vi "Message Based DAQ.vi"() -> ()   [LabVIEW 2014]
uses:
  <vilib>/Utility/error.llb/DialogType.ctl
  vilib/Message/Msg Post UI Message.vi
  vilib/Message/Msg Post Queue Message.vi
  vilib/Message/Msg Send Queue Message.vi
panel:
  in  "File Path":path
  in  "Acquire Data":bool
  in  "Log Data":bool
  in  "File Comment":string
  in  "DAQ Parameters":T1={"physical channels"="", "maximum value"=5.0, "minimum value"=-5.0, "rate"=1000.0, "read period"=0.5} {"read period" format="%0.2f"; "rate" format="%0.2f"; "minimum value" format="%0.2f"; "maximum value" format="%0.2f"}
  out "Waveform Chart":waveform(dbl)(graph)
  in  "quit":bool
  # "V"
  # "V"
  # "Hz"
  # "s"
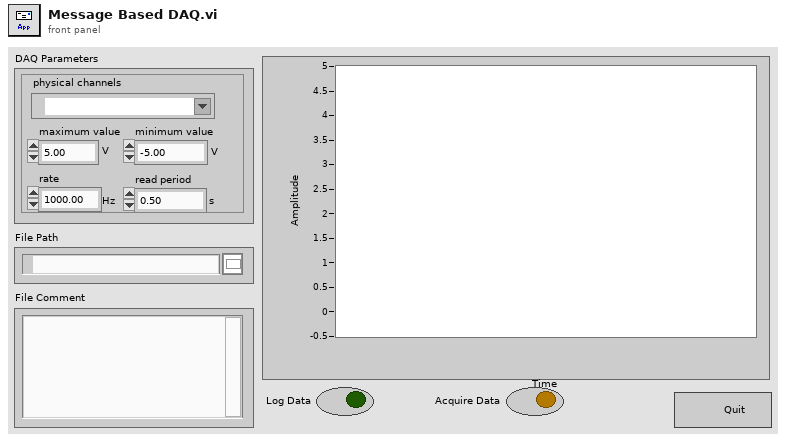
[diagram p1: front panel]
types:
  T1 = cluster{"physical channels":tag, "maximum value":dbl, "minimum value":dbl, "rate":dbl, "read period":dbl}
  T2 = typedef "DialogType.ctl" = u16
  T3 = enum16{"Left Button", "Center Button", "Right Button", "Window Close"}
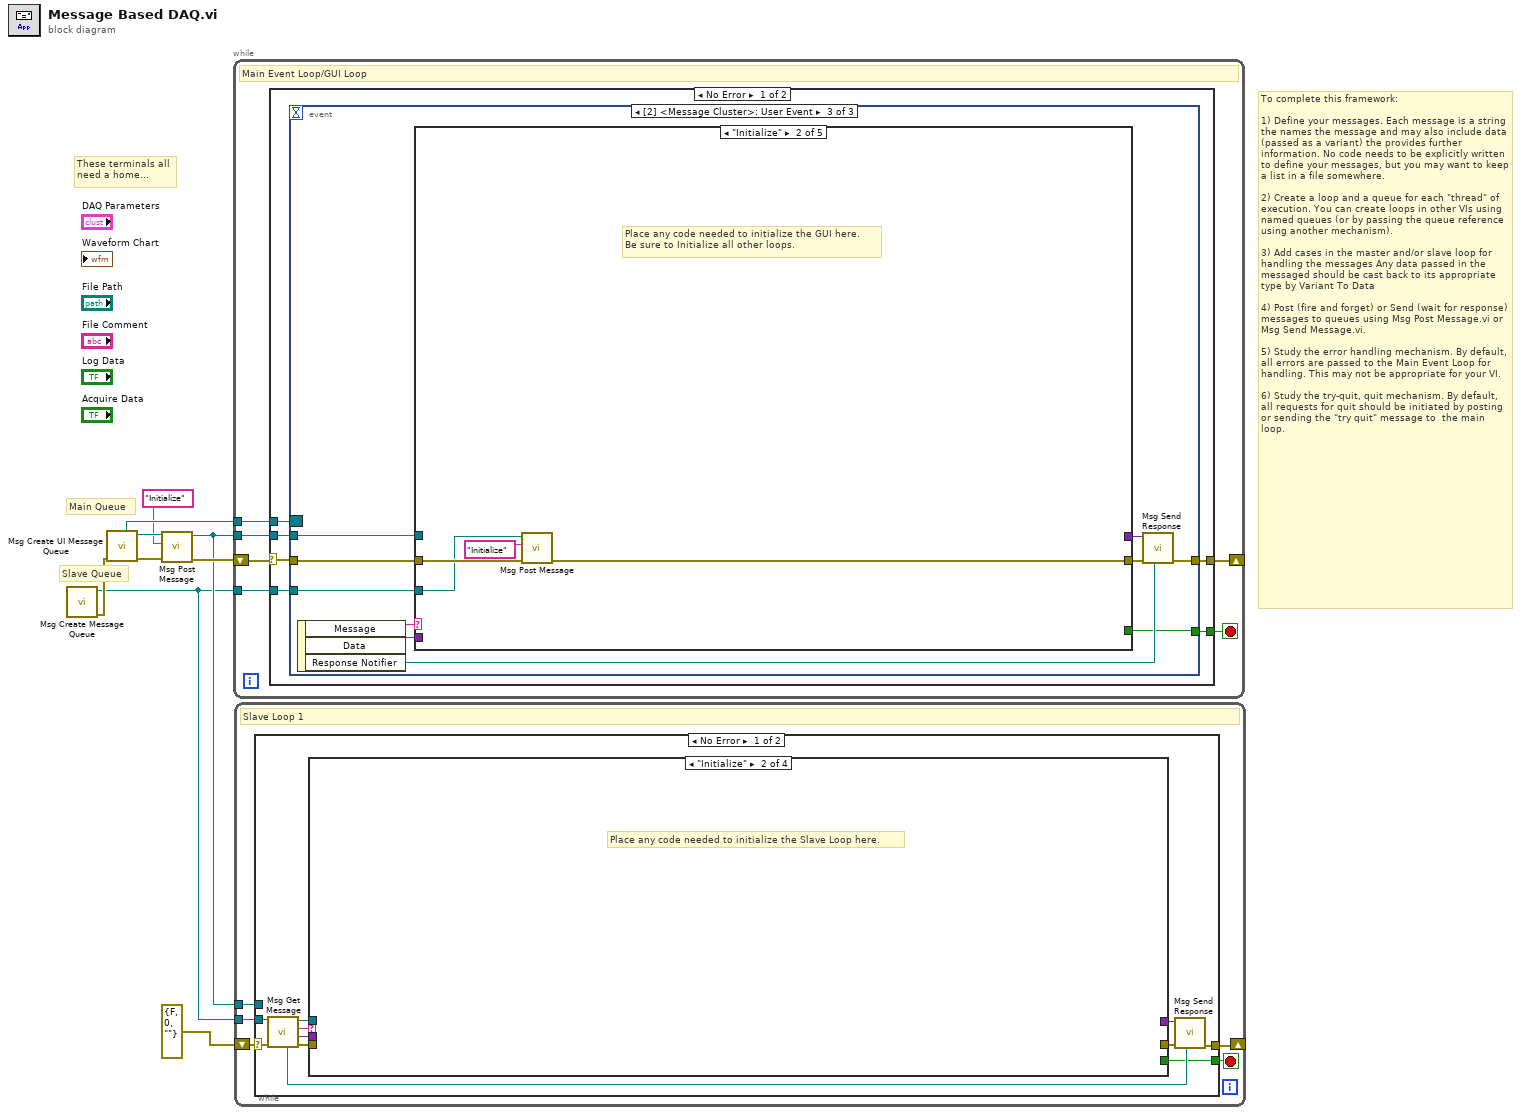
[diagram p0: block diagram]
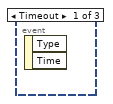
[diagram p2: hidden frame]
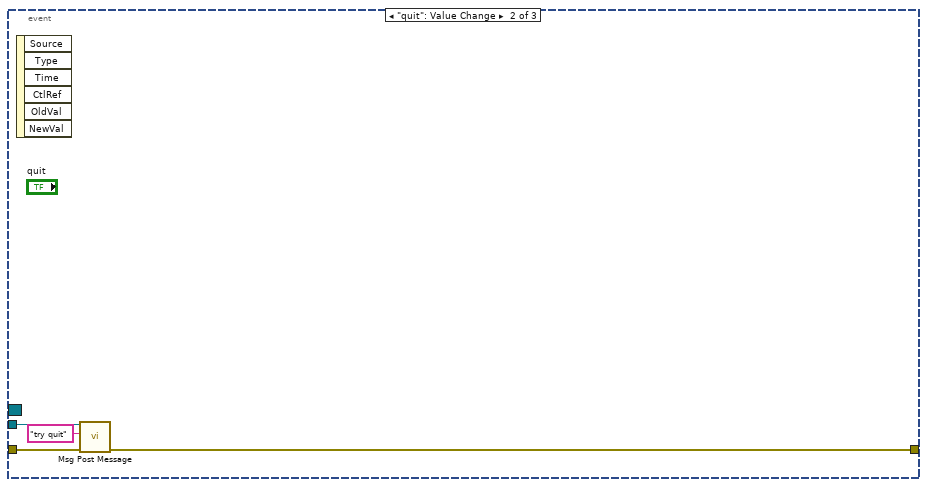
[diagram p3: hidden frame]
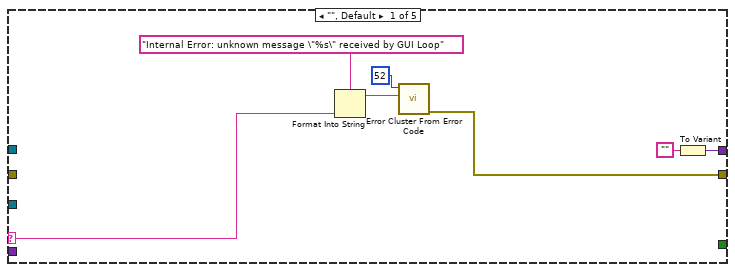
[diagram p4: hidden frame]
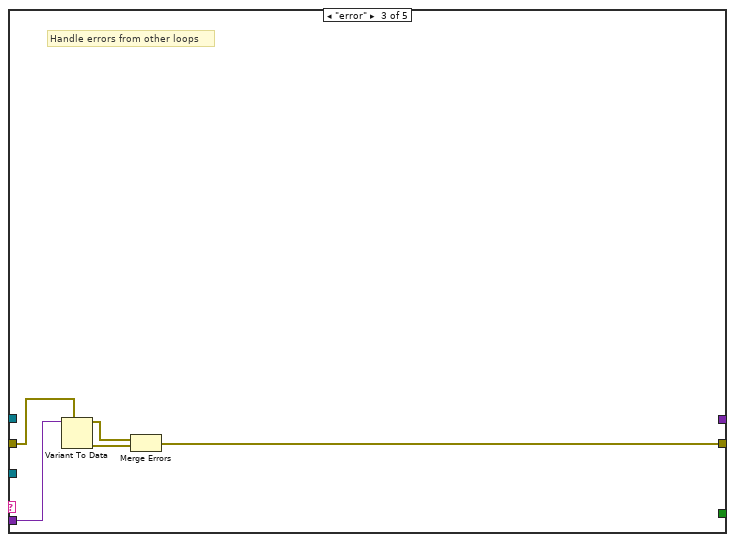
[diagram p5: hidden frame]
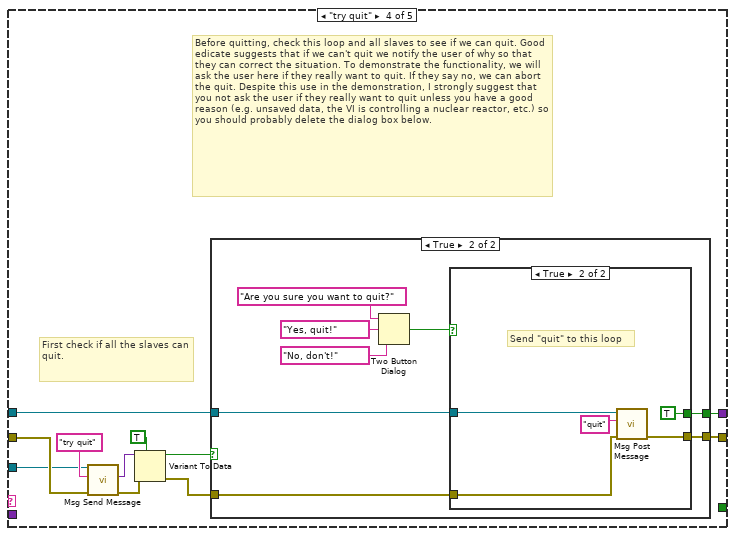
[diagram p6: hidden frame]
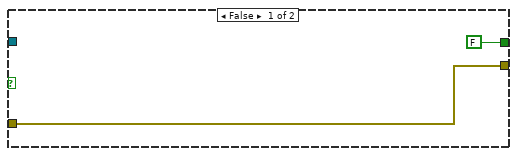
[diagram p7: hidden frame]
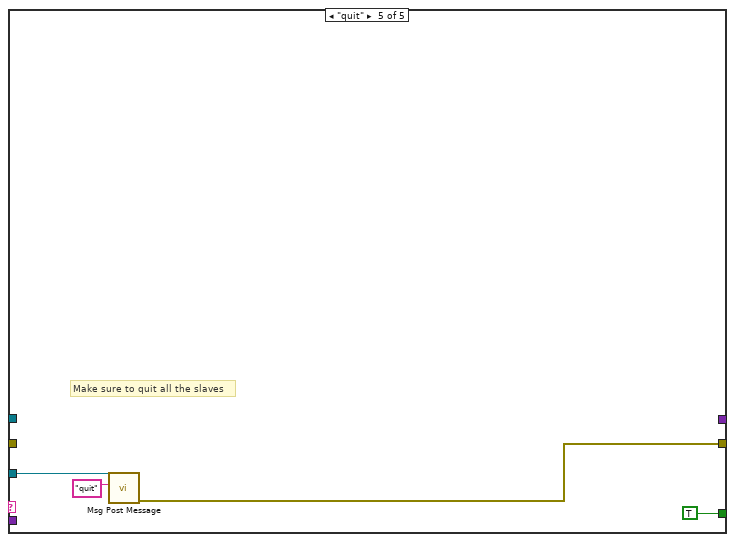
[diagram p9: hidden frame]
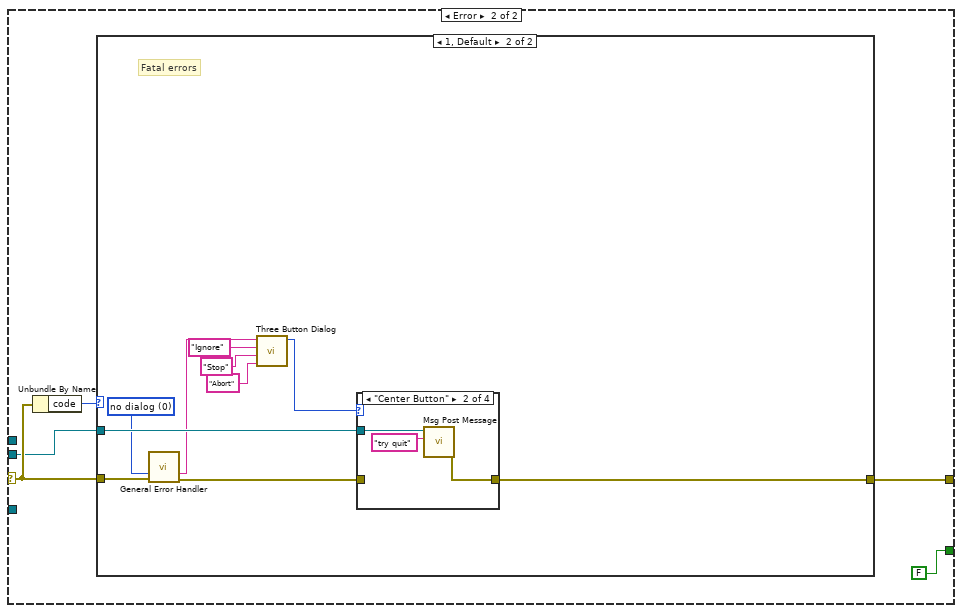
[diagram p10: hidden frame]
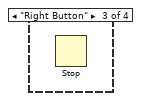
[diagram p13: hidden frame]
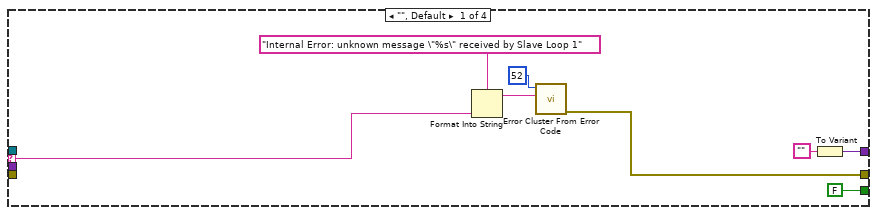
[diagram p15: hidden frame]
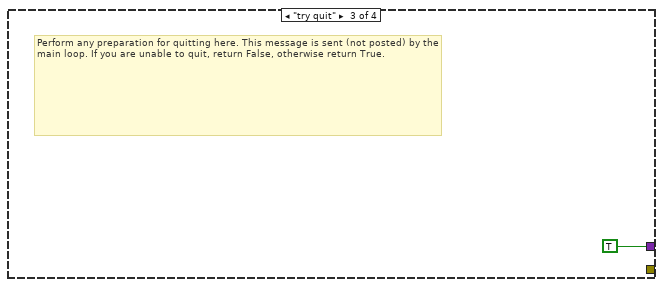
[diagram p16: hidden frame]
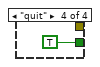
[diagram p17: hidden frame]
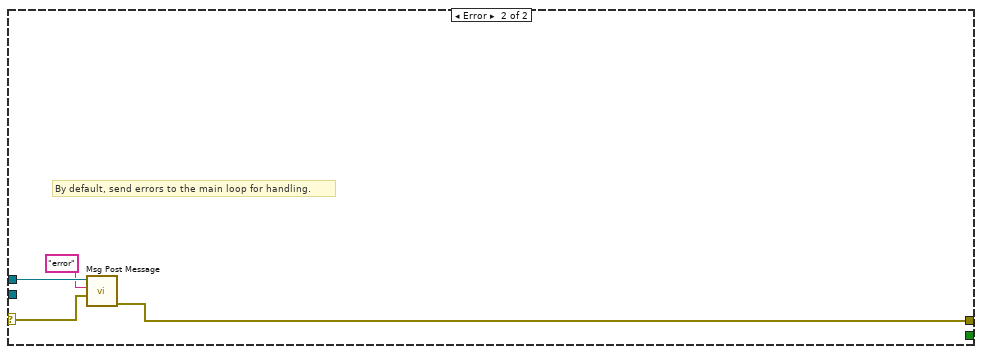
[diagram p18: hidden frame]
diagram:
  # "These terminals all\nneed a home..."
  # "To complete this framework:\n\n1) Define your messages. Each message is a string the names the message and may also include data (passed as a variant) the provides further information. No code needs to be explicitly written to define your messages, but you may want to keep a list in a file somewhere.\n\n2) Create a loop and a queue for each \"thread\" of execution. You can create loops in other VIs using named queues (or by passing the queue reference using another mechanism).\n\n3) Add cases in the master and/or slave loop for handling the messages Any data passed in the messaged should be cast back to its appropriate type by Variant To Data\n\n4) Post (fire and forget) or Send (wait for response) messages to queues using Msg Post Message.vi or Msg Send Message.vi.\n\n5) Study the error handling mechanism. By default, all errors are passed to the Main Event Loop for handling. This may not be appropriate for your VI.\n\n6) Study the try-quit, quit mechanism. By default, all requests for quit should be initiated by posting or sending the \"try quit\" message to  the main loop."
  # "Main Queue"
  # "Slave Queue"
  n1 = call "Msg Create Message Queue.vi"() -> ("error out"=w5:errorcluster, "queue out"=w2:refnum<queue>)  [unwired: 7 in, 1 out]
  n2 = call "Msg Create UI Message Queue.vi"("error in (no error)"=w5) -> ("error out"=w6:errorcluster, "user event"=w8:refnum<user-event>, "Event Registration Refnum out"=w9:refnum<event-registration>)  [unwired: 6 in]
  n3 = call-poly "Msg Post Message.vi"("error in (no error)"=w6, "Message"="Initialize", "user event"=w8) -> ("error out"=w4:errorcluster, "user event out"=w3:refnum<user-event>)  [unwired: 4 in, 1 out]
  n4 = while {
    tunnel: w9 -> [w14]
    shift-right: [w12] -> _
    shift-left: w4 -> [w10]
    tunnel: w3 -> [w13]
    tunnel: w2 -> [w11]
    stop <- w15 stop-if-true
    # "Main Event Loop/GUI Loop"
    n5 = case shown="No Error" w10 {
      selector: w10 -> [w16 w85]
      tunnel: [w21 FALSE] -> w15
      tunnel: w14 -> [w20 _]
      tunnel: w13 -> [w19 w84]
      tunnel: [w18 w83] -> w12
      tunnel: w11 -> [w17 _]
      frame No Error {
        n6 = event shown="[2] <Message Cluster>: User Event" {
          selector: w20 -> [_ _ _]
          dyn-events: _ -> [_ _ _]
          timeout: _ -> [_ _ _]
          tunnel: [_ _ w26] -> w21
          tunnel: w19 -> [_ w25 w27]
          tunnel: w16 -> [_ w24 w32]
          tunnel: [_ w23 w30] -> w18
          tunnel: w17 -> [_ _ w28]
          event Timeout {
            n7 = event-data() -> ()  [unwired: 1 in, 2 out]
          }
          event "quit": Value Change {
            n8 = event-data() -> ()  [unwired: 1 in, 6 out]
            n9 = call-poly "Msg Post Message.vi"("error in (no error)"=w24, "Message"="try quit", "user event"=w25) -> ("error out"=w23:errorcluster)  [unwired: 4 in, 2 out]
          }
          event User Event {
            n10 = event-data() -> ("Message"=w35:string, "Data"=w29:variant, "Response Notifier"=w33:refnum<notifier>)  [unwired: 1 in]
            n11 = case shown="\"Initialize\"" w35 {
              selector: w35 -> [w40 _ _ _ _]
              tunnel: [w41 _ _ w55 _] -> w34
              tunnel: w32 -> [_ w46 w50 w62 _]
              tunnel: [w36 w43 w47 w56 w79] -> w31
              tunnel: w29 -> [_ _ w51 _ _]
              tunnel: w28 -> [_ w45 _ w53 w80]
              tunnel: w27 -> [_ _ _ w57 _]
              tunnel: [_ _ _ _ TRUE] -> w26
              frame "", Default {
                n12 = Format Into String(format string="Internal Error: unknown message \"%s\" received by GUI Loop" ("error message (\"\")"), w40) -> (resulting string=w37:string)  [unwired: 2 in, 1 out]
                n13 = call <vilib>:"Error Cluster From Error Code.vi"("error message (\"\")"=w37, "error code (0)"=52) -> ("error out"=w36:errorcluster)  [unwired: 7 in]
                n14 = To Variant(anything="") -> (Variant=w41:variant)
              }
              frame "Initialize" {
                # "Place any code needed to initialize the GUI here. \nBe sure to Initialize all other loops."
                n15 = call-poly "Msg Post Message.vi"("error in (no error)"=w46, "Message"="Initialize", "queue"=w45) -> ("error out"=w43:errorcluster)  [unwired: 4 in, 2 out]
              }
              frame "error" {
                # "Handle errors from other loops"
                n16 = Variant To Data(type=w50, Variant=w51) -> (data=w49:errorcluster, error out=w48:errorcluster)  [unwired: 1 in]
                n17 = Merge Errors(w49, w48) -> (w47:errorcluster)
              }
              frame "try quit" {
                # "Before quitting, check this loop and all slaves to see if we can quit. Good edicate suggests that if we can't quit we notify the user of why so that they can correct the situation. To demonstrate the functionality, we will ask the user here if they really want to quit. If they say no, we can abort the quit. Despite this use in the demonstration, I strongly suggest that you not ask the user if they really want to quit unless you have a good reason (e.g. unsaved data, the VI is controlling a nuclear reactor, etc.) so you should probably delete the dialog box below."
                # "First check if all the slaves can quit."
                n18 = call-poly "Msg Send Message.vi"("error in (no error)"=w62, "Message"="try quit", "queue"=w53) -> ("error out"=w60:errorcluster, "response"=w54:variant)  [unwired: 3 in, 2 out]
                n19 = Variant To Data(error in=w60, type=TRUE, Variant=w54) -> (data=w52:bool, error out=w58:errorcluster)
                n20 = case shown="True" w52 {
                  tunnel: w58 -> [w64 w71]
                  tunnel: w57 -> [_ w72]
                  tunnel: [w64 w70] -> w56
                  tunnel: [FALSE w69] -> w55
                  frame False {
                  }
                  frame True {
                    n21 = Two Button Dialog(message="Are you sure you want to quit?", 1:"No, don't!" ("T button name (\"OK\")"), 2:"Yes, quit!" ("T button name (\"OK\")")) -> (T button?=w65:bool)
                    n22 = case shown="True" w65 {
                      tunnel: w72 -> [_ w78]
                      tunnel: w71 -> [w73 w76]
                      tunnel: [w73 w75] -> w70
                      tunnel: [_ TRUE] -> w69
                      frame False {
                      }
                      frame True {
                        # "Send \"quit\" to this loop"
                        n23 = call-poly "Msg Post Message.vi"("error in (no error)"=w76, "Message"="quit", "user event"=w78) -> ("error out"=w75:errorcluster)  [unwired: 4 in, 2 out]
                      }
                    }
                  }
                }
              }
              frame "quit" {
                # "Make sure to quit all the slaves"
                n24 = call-poly "Msg Post Message.vi"("Message"="quit", "queue"=w80) -> ("error out"=w79:errorcluster)  [unwired: 5 in, 2 out]
              }
            }
            n25 = call "Msg Send Response.vi"("Response Notifier"=w33, "error in (no error)"=w31, "response"=w34) -> ("error out"=w30:errorcluster)  [unwired: 6 in]
          }
        }
      }
      frame Error {
        n26 = Unbundle By Name(w85) -> ("code"=w86:i32)
        n27 = case shown="1, Default" w86 {
          tunnel: w85 -> [_ w97]
          tunnel: w84 -> [_ w96]
          tunnel: [_ w94] -> w83
          frame 0 {
            # "Ignore these errors"
          }
          frame 1, Default {
            w93 = T2 0 items=["no dialog", "OK message", "continue or stop message", "OK message + warnings", "continue/stop + warnings"] ("type of dialog (OK msg:1)")
            # "Fatal errors"
            n28 = call <vilib>:"General Error Handler.vi"("type of dialog (OK msg:1)"=w93, "error in (no error)"=w97) -> ("message"=w92:string, "error out"=w95:errorcluster)  [unwired: 9 in, 3 out]
            n29 = call <vilib>:"Three Button Dialog.vi"("Right Button Text (\"Cancel\")"="Abort" ("Right Button Text (\"Cancel\")"), "Center Button Text (\"No\")"="Stop" ("Center Button Text (\"No\")"), "Left Button Text (\"Yes\")"="Ignore" ("Left Button Text (\"Yes\")"), "message"=w92) -> ("Which Button?"=w88:T3)  [unwired: 7 in]
            n30 = case shown="\"Center Button\"" w88 {
              tunnel: w96 -> [_ w100 _ _]
              tunnel: w95 -> [_ _ _ _]
              tunnel: [_ w98 _ _] -> w94
              frame "Left Button", Default {
              }
              frame "Center Button" {
                n31 = call-poly "Msg Post Message.vi"("Message"="try quit", "user event"=w100) -> ("error out"=w98:errorcluster)  [unwired: 5 in, 2 out]
              }
              frame "Right Button" {
                n32 = Stop() -> ()  [unwired: 1 in]
              }
              frame "Window Close" {
              }
            }
          }
        }
      }
    }
  }
  n33 = while {
    tunnel: w3 -> [w101]
    tunnel: w2 -> [w105]
    shift-right: [w104] -> _
    shift-left: errorcluster {"status"=FALSE, "code"=0, "source"=""} ("error out") -> [w102]
    stop <- w103 stop-if-true
    # "Slave Loop 1"
    n34 = case shown="No Error" w102 {
      selector: w102 -> [w106 w128]
      tunnel: w105 -> [w116 _]
      tunnel: [w110 w127] -> w104
      tunnel: [w107 _] -> w103
      tunnel: w101 -> [_ w130]
      frame No Error {
        n35 = call "Msg Get Message.vi"("queue"=w116, "error in (no error)"=w106) -> ("Response Notifier"=w109:refnum<notifier>, "queue out"=w112:refnum<queue>, "Message"=w114:string, "Data"=w113:variant, "error out"=w115:errorcluster)  [unwired: 2 in]
        n36 = case shown="\"Initialize\"" w114 {
          selector: w114 -> [w117 _ _ _]
          tunnel: [w118 _ _ _] -> w111
          tunnel: w115 -> [_ _ _ _]
          tunnel: w113 -> [_ _ _ _]
          tunnel: w112 -> [_ _ _ _]
          tunnel: [w123 _ TRUE _] -> w108
          tunnel: [FALSE _ _ TRUE] -> w107
          frame "", Default {
            n37 = Format Into String(format string="Internal Error: unknown message \"%s\" received by Slave Loop 1" ("error message (\"\")"), w117) -> (resulting string=w121:string)  [unwired: 2 in, 1 out]
            n38 = call <vilib>:"Error Cluster From Error Code.vi"("error message (\"\")"=w121, "error code (0)"=52) -> ("error out"=w118:errorcluster)  [unwired: 7 in]
            n39 = To Variant(anything="") -> (Variant=w123:variant)
          }
          frame "Initialize" {
            # "Place any code needed to initialize the Slave Loop here."
          }
          frame "try quit" {
            # "Perform any preparation for quitting here. This message is sent (not posted) by the main loop. If you are unable to quit, return False, otherwise return True."
          }
          frame "quit" {
          }
        }
        n40 = call "Msg Send Response.vi"("Response Notifier"=w109, "error in (no error)"=w111, "response"=w108) -> ("error out"=w110:errorcluster)  [unwired: 6 in]
      }
      frame Error {
        # "By default, send errors to the main loop for handling."
        n41 = call-poly "Msg Post Message.vi"("Data"=w128, "Message"="error", "user event"=w130) -> ("error out"=w127:errorcluster)  [unwired: 4 in, 2 out]
      }
    }
  }
